vi "Initialize Attributes.vi"(8 "error in (no error)":errorcluster, 10 "Attribute Data":variant, 11 "CS++IEFWerner in":refnum<class "CS++IEFWerner.lvclass">) -> (0 "error out":errorcluster, 2 "Found?":bool, 3 "CS++IEFWerner out":refnum<class "CS++IEFWerner.lvclass">)   [LabVIEW 2015, in "CS++IEFWerner.lvlib" / "CS++IEFWerner.lvclass"]
doc: "Initialize object attribute.\n\nUnique resources should be allocated elsewhere!"
uses:
  CS++IEFWerner.lvclass
  CSPP_Core/Classes/CS++ProcessVariables/ProcessVariable/PV.lvclass
  CSPP_Core/Actors/CS++BaseActor/CS++BaseActor.lvclass/CS++BaseActor.ctl
  CSPP_Core/Actors/CS++DeviceActor/CS++DeviceActor.lvclass/CS++DeviceActor.ctl
  CSPP_Core/Classes/CS++ProcessVariables/ProcessVariable/PV.lvclass/PV.ctl
  CS++IEFWerner.lvclass/CS++IEFWerner.ctl
  CSPP_Core/Classes/CS++ProcessVariables/ProcessVariable/Write PV URL.vi
  CSPP_Core/Classes/CS++ProcessVariables/ProcessVariable/Write Type Descriptor.vi
  <vilib>/Utility/error.llb/Error Cluster From Error Code.vi
  CSPP_DeviceBase/CS++Motor/CS++Motor.lvclass
  CSPP_Core/Classes/CS++BaseClasses/Factory/CS++Factory.lvclass
  CSPP_Core/Libraries/Utilities/CS++Utilities.lvlib
  CSPP_Core/Classes/CS++ProcessVariables/CS++ProcessVariables.lvlib
  CSPP_Core/Actors/CS++BaseActor/CS++BaseActor.lvclass
  CSPP_Core/Actors/CS++DeviceActor/CS++DeviceActor.lvclass
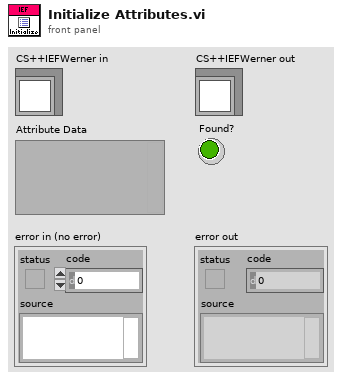
[diagram p1: front panel]
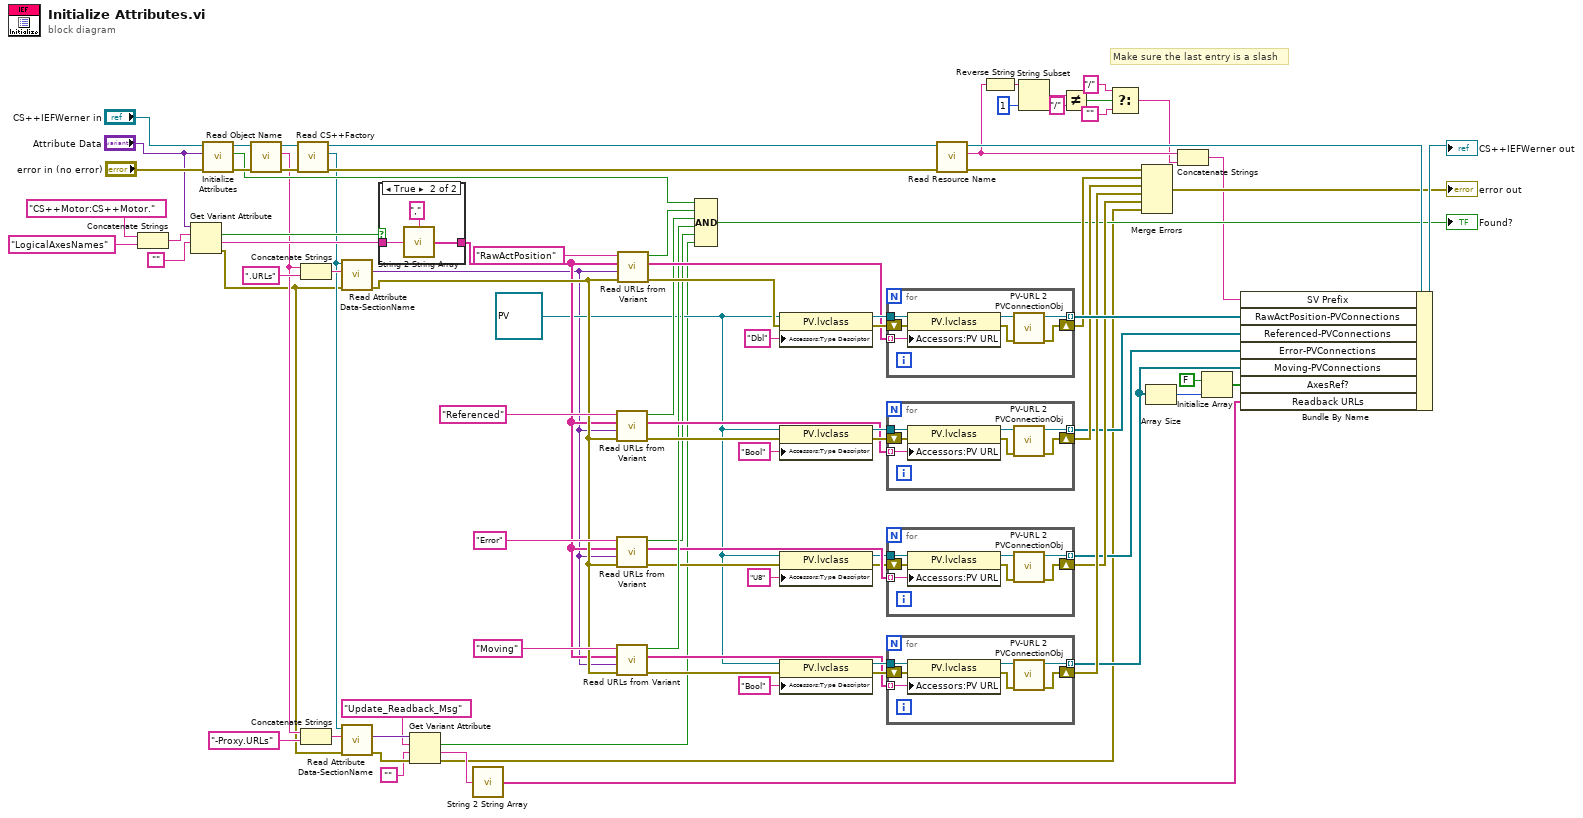
[diagram p0: block diagram]
diagram:
  w36 = refnum<class "PV.lvclass"> refnum ("CS++ProcessVariables.lvlib:PV.lvclass")
  # "Make sure the last entry is a slash"
  n1 = Concatenate Strings("CS++Motor:CS++Motor.", "LogicalAxesNames" ("string")) -> (w85:string)
  n2 = Get Variant Attribute(Variant="Attribute Data", name=w85, default value (empty Variant)="") -> (found=w82:bool, value=w83:string, error out=w9:errorcluster)  [unwired: 1 in, 1 out]
  n3 = call-parent "Initialize Attributes.vi"("error in (no error)"="error in (no error)", "Attribute Data"="Attribute Data", "CS++Motor in"="CS++IEFWerner in") -> ("error out"=w33:errorcluster, "Found?"=w32:bool, "CS++Motor out"=w34:refnum<class "CS++IEFWerner.lvclass">)  [unwired: 6 in]
  n4 = call "Read Object Name.vi"("error in (no error)"=w33, "CS++BaseActor in"=w34) -> ("error out"=w71:errorcluster, "Object Name"=w12:string, "CS++BaseActor out"=w72:refnum<class "CS++IEFWerner.lvclass">)  [unwired: 7 in]
  n5 = call "Read CS++Factory.vi"("error in (no error)"=w71, "CS++BaseActor in"=w72) -> ("error out"=w40:errorcluster, "CS++Factory"=w10:refnum<class "CS++Factory.lvclass">, "CS++BaseActor out"=w42:refnum<class "CS++IEFWerner.lvclass">)  [unwired: 7 in]
  n6 = Concatenate Strings(w12, ".URLs" ("string")) -> (w70:string)
  n7 = Concatenate Strings(w12, "-Proxy.URLs" ("string")) -> (w11:string)
  n8 = call-dynamic "Read Attribute Data-SectionName.vi"("error in (no error)"=w9, "Object Name"=w70, "CS++Factory in"=w10) -> ("error out"=w38:errorcluster, "Attribute Data"=w35:variant)  [unwired: 6 in, 1 out]
  n9 = call-dynamic "Read Attribute Data-SectionName.vi"("error in (no error)"=w9, "Object Name"=w11, "CS++Factory in"=w10) -> ("error out"=w7:errorcluster, "Attribute Data"=w8:variant)  [unwired: 6 in, 1 out]
  n10 = case shown="True" w82 {
    tunnel: w83 -> [_ w92]
    tunnel: [_ w91] -> w37
    frame False {
    }
    frame True {
      n11 = call "String 2 String Array.vi"("String"=w92, "Delimiter (\",\")"="," ("Delimiter (\",\")")) -> ("Substrings"=w91:string[])
    }
  }
  n12 = Get Variant Attribute(Variant=w8, name="Update_Readback_Msg", default value (empty Variant)="", error in=w7) -> (found=w4:bool, value=w3:string, error out=w2:errorcluster)  [unwired: 1 out]
  n13 = call "String 2 String Array.vi"("String"=w3) -> ("Substrings"=w1:string[])  [unwired: 1 in]
  n14 = call "Read URLs from Variant.vi"("Error In"=w38, "URL Section Data"=w35, "Channel Names"=w37, "URL Prefix"="Referenced") -> ("Error Out"=w67:errorcluster, "URLs"=w64:string[], "Found?"=w45:bool)  [unwired: 4 in, 1 out]
  n15 = call "Read URLs from Variant.vi"("Error In"=w38, "URL Section Data"=w35, "Channel Names"=w37, "URL Prefix"="Error") -> ("Error Out"=w53:errorcluster, "URLs"=w52:string[], "Found?"=w48:bool)  [unwired: 4 in, 1 out]
  n16 = call "Read URLs from Variant.vi"("Error In"=w38, "URL Section Data"=w35, "Channel Names"=w37, "URL Prefix"="Moving") -> ("Error Out"=w58:errorcluster, "URLs"=w59:string[], "Found?"=w57:bool)  [unwired: 4 in, 1 out]
  n17 = call "Read URLs from Variant.vi"("Error In"=w38, "URL Section Data"=w35, "Channel Names"=w37, "URL Prefix"="RawActPosition") -> ("Error Out"=w76:errorcluster, "URLs"=w77:string[], "Found?"=w81:bool)  [unwired: 4 in, 1 out]
  n18 = Compound Arithmetic op=AND(w32, w81, w45, w57, w48, w4) -> (→"Found?":bool)
  n19 = property class="PV.lvclass"(reference=w36, error in=w76, "Accessors:Type Descriptor"="Dbl" ("Type Descriptor")) -> (reference out=w79:refnum<class "PV.lvclass">, error out=w78:errorcluster)
  n20 = property class="PV.lvclass"(reference=w36, error in=w67, "Accessors:Type Descriptor"="Bool" ("Type Descriptor")) -> (reference out=w66:refnum<class "PV.lvclass">, error out=w65:errorcluster)
  n21 = property class="PV.lvclass"(reference=w36, error in=w53, "Accessors:Type Descriptor"="U8" ("Type Descriptor")) -> (reference out=w51:refnum<class "PV.lvclass">, error out=w50:errorcluster)
  n22 = property class="PV.lvclass"(reference=w36, error in=w58, "Accessors:Type Descriptor"="Bool" ("Type Descriptor")) -> (reference out=w60:refnum<class "PV.lvclass">, error out=w61:errorcluster)
  n23 = for {
    tunnel: w79 -> [w98]
    tunnel: w77 -> [w97] mode=indexing
    tunnel: [w96] -> w74 mode=indexing
    shift-right: [w95] -> w73
    shift-left: w78 -> [w93]
    n24 = property class="PV.lvclass"(reference=w98, error in=w93, "Accessors:PV URL"=w97) -> (reference out=w99:refnum<class "PV.lvclass">, error out=w94:errorcluster)
    n25 = call "PV-URL 2 PVConnectionObj.vi"("Error In"=w94, "PV"=w99) -> ("Error Out"=w95:errorcluster, "PVConnection"=w96:refnum<class "PVConnection.lvclass">)  [unwired: 7 in, 1 out]
  }
  n26 = for {
    tunnel: w66 -> [w105]
    tunnel: w64 -> [w104] mode=indexing
    tunnel: [w103] -> w44 mode=indexing
    shift-right: [w102] -> w63
    shift-left: w65 -> [w100]
    n27 = property class="PV.lvclass"(reference=w105, error in=w100, "Accessors:PV URL"=w104) -> (reference out=w106:refnum<class "PV.lvclass">, error out=w101:errorcluster)
    n28 = call "PV-URL 2 PVConnectionObj.vi"("Error In"=w101, "PV"=w106) -> ("Error Out"=w102:errorcluster, "PVConnection"=w103:refnum<class "PVConnection.lvclass">)  [unwired: 7 in, 1 out]
  }
  n29 = for {
    tunnel: w51 -> [w112]
    tunnel: w52 -> [w111] mode=indexing
    tunnel: [w110] -> w43 mode=indexing
    shift-right: [w109] -> w47
    shift-left: w50 -> [w107]
    n30 = property class="PV.lvclass"(reference=w112, error in=w107, "Accessors:PV URL"=w111) -> (reference out=w113:refnum<class "PV.lvclass">, error out=w108:errorcluster)
    n31 = call "PV-URL 2 PVConnectionObj.vi"("Error In"=w108, "PV"=w113) -> ("Error Out"=w109:errorcluster, "PVConnection"=w110:refnum<class "PVConnection.lvclass">)  [unwired: 7 in, 1 out]
  }
  n32 = for {
    tunnel: w60 -> [w119]
    tunnel: w59 -> [w118] mode=indexing
    tunnel: [w117] -> w25 mode=indexing
    shift-right: [w116] -> w55
    shift-left: w61 -> [w114]
    n33 = property class="PV.lvclass"(reference=w119, error in=w114, "Accessors:PV URL"=w118) -> (reference out=w120:refnum<class "PV.lvclass">, error out=w115:errorcluster)
    n34 = call "PV-URL 2 PVConnectionObj.vi"("Error In"=w115, "PV"=w120) -> ("Error Out"=w116:errorcluster, "PVConnection"=w117:refnum<class "PVConnection.lvclass">)  [unwired: 7 in, 1 out]
  }
  n35 = call "Read Resource Name.vi"("error in (no error)"=w40, "CS++DeviceActor in"=w42) -> ("error out"=w39:errorcluster, "Resource Name"=w16:string, "CS++DeviceActor out"=w41:refnum<class "CS++IEFWerner.lvclass">)  [unwired: 7 in]
  n36 = Reverse String(1:w16) -> (0:w23:string)
  n37 = String Subset(string=w23, length (rest)=1 ("length (rest)")) -> (substring=w21:string)  [unwired: 1 in]
  n38 = Not Equal?(x=w21, y="/") -> (x != y?=w19:bool)
  n39 = Select(t="/" ("y"), s=w19, f="") -> (s? t:f=w14:string)
  n40 = Merge Errors(w39, w73, w63, w55, w47, w2) -> (→"error out":errorcluster)
  n41 = Array Size(array=w25) -> (size(s)=w24:i32)
  n42 = Concatenate Strings(w16, w14) -> (w15:string)
  n43 = Initialize Array(FALSE, w24) -> (w27:bool[])
  n44 = Bundle By Name(cluster=w41, "SV Prefix"=w15, "RawActPosition-PVConnections"=w74, "Referenced-PVConnections"=w44, "Error-PVConnections"=w43, "Moving-PVConnections"=w25, "AxesRef?"=w27, "Readback URLs"=w1) -> (→"CS++IEFWerner out":refnum<class "CS++IEFWerner.lvclass">)
